vi "getPictureTypeAndName.vi"(8 "error in (no error)":errorcluster, 11 "xwpfRun.Figure in":refnum<class "xwpfRun.Figure.lvclass">) -> (0 "error out":errorcluster, 3 "xwpfRun.Figure out":refnum<class "xwpfRun.Figure.lvclass">)   [LabVIEW 2017, in "Word_Specific.lvlib" / "xwpfRun.Figure.lvclass"]
uses:
  xwpfRun.Figure.lvclass
  xwpfRun.Figure.lvclass/xwpfRun.Figure.ctl
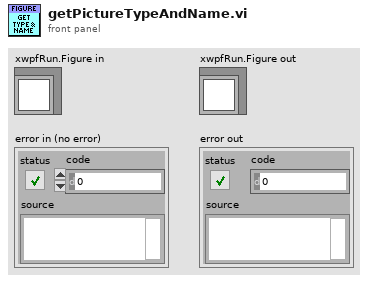
[diagram p1: front panel]
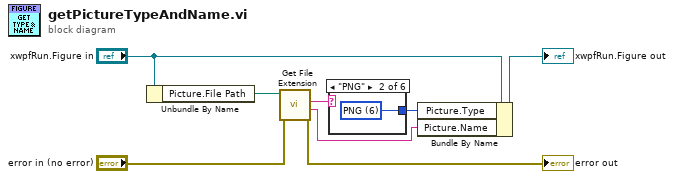
[diagram p0: block diagram]
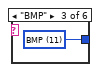
[diagram p3: hidden frame]
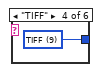
[diagram p4: hidden frame]
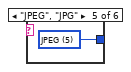
[diagram p5: hidden frame]
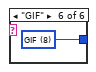
[diagram p6: hidden frame]
diagram:
  n1 = Unbundle By Name("xwpfRun.Figure in") -> ("Picture.File Path"=w7:path)
  n2 = call <vilib>:"Get File Extension.vi"("error in (no error)"="error in (no error)", "file"=w7) -> ("error out"=→"error out":errorcluster, "filename without extension"=w8:string, "lowercase file extension"=w2:string)  [unwired: 5 in, 2 out]
  n3 = case shown="\"PNG\"" w2 {
    tunnel: [_ w9 w10 w11 w12 w13] -> w1
    frame "False", Default {
    }
    frame "PNG" {
      w9 = 6 items=["BMP"=11, "DIB"=7, "EMF"=2, "EPS"=10, "GIF"=8, "JPEG"=5, "PICT"=4, "PNG"=6, "TIFF"=9, "WMF"=3, "WPG"=12] ("PictureType")
    }
    frame "BMP" {
      w10 = 11 items=["BMP"=11, "DIB"=7, "EMF"=2, "EPS"=10, "GIF"=8, "JPEG"=5, "PICT"=4, "PNG"=6, "TIFF"=9, "WMF"=3, "WPG"=12] ("PictureType")
    }
    frame "TIFF" {
      w11 = 9 items=["BMP"=11, "DIB"=7, "EMF"=2, "EPS"=10, "GIF"=8, "JPEG"=5, "PICT"=4, "PNG"=6, "TIFF"=9, "WMF"=3, "WPG"=12] ("PictureType")
    }
    frame "JPEG", "JPG" {
      w12 = 5 items=["BMP"=11, "DIB"=7, "EMF"=2, "EPS"=10, "GIF"=8, "JPEG"=5, "PICT"=4, "PNG"=6, "TIFF"=9, "WMF"=3, "WPG"=12] ("PictureType")
    }
    frame "GIF" {
      w13 = 8 items=["BMP"=11, "DIB"=7, "EMF"=2, "EPS"=10, "GIF"=8, "JPEG"=5, "PICT"=4, "PNG"=6, "TIFF"=9, "WMF"=3, "WPG"=12] ("PictureType")
    }
  }
  n4 = Bundle By Name(cluster="xwpfRun.Figure in", "Picture.Type"=w1, "Picture.Name"=w8) -> (→"xwpfRun.Figure out":refnum<class "xwpfRun.Figure.lvclass">)
